vi "AOL Z Cal load-Load handler.vi"(11 "Loaded file":refnum<vi>) -> ()   [LabVIEW 2013]
uses:
  Typedefs/Which path.ctl
  Typedefs/Read Write Enum.ctl
  Typedefs/Functional global standard states.ctl
  Configuration code/Calibration/Globals/gl_Calibration globals.vi
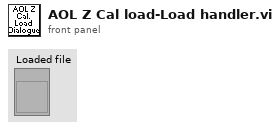
[diagram p1: front panel]
types:
  T1 = typedef "Which path.ctl" = enum16{"Configuration Files", "Calibration Files", "Images", "Setup.ini", "Loaded User profile.ini", "User's-Previous session.ini", "New user profile.ini", "Selected User profile.ini", "User profiles folder", "Power meter scaling.txt", "FOV Cal.ini"}
  T2 = typedef "Read Write Enum.ctl" = enum16{"Read", "Write"}
  T3 = typedef "Functional global standard states.ctl" = enum16{"Initialise", "Read", "Write", "Load", "Save", "Clear"}
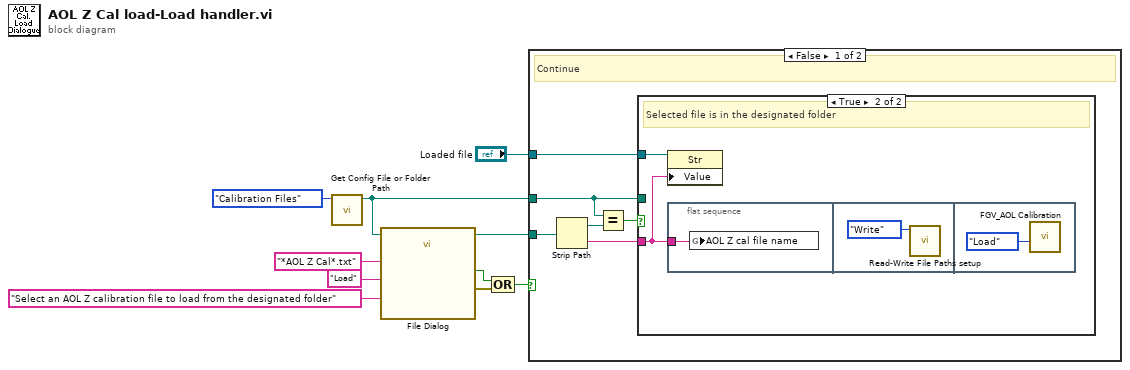
[diagram p0: block diagram]
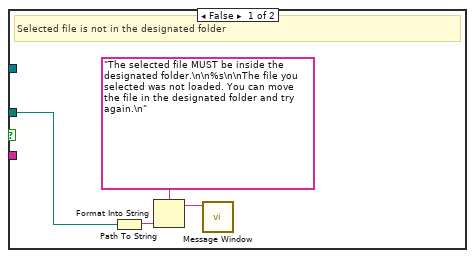
[diagram p2: hidden frame]
diagram:
  n1 = call "Get Config File or Folder Path.vi"("Which file or folder?"=Which_path."Calibration Files" ("Which file?")) -> ("File Path"=w2:path)  [unwired: 8 in, 2 out]
  n2 = call "File Dialog"("start path"=w2, "prompt"="Select an AOL Z calibration file to load from the designated folder", "button label"="Load", "pattern (all files)"="*AOL Z Cal*.txt") -> ("selected path"=w3:path, "cancelled"=w8:bool, "error out"=w7:errorcluster)  [unwired: 8 in, 1 out]
  n3 = Compound Arithmetic op=OR(w8, w7) -> (w6:bool)
  n4 = case shown="False" w6 {
    tunnel: w3 -> [w16 _]
    tunnel: w2 -> [w12 _]
    tunnel: "Loaded file" -> [w11 _]
    frame False {
      # "Continue"
      n5 = Strip Path(path=w16) -> (stripped path=w14:path, name=w15:string)
      n6 = Equal?(x=w12, y=w14) -> (x = y?=w13:bool)
      n7 = case shown="True" w13 {
        tunnel: w15 -> [_ w21]
        tunnel: w12 -> [w17 _]
        tunnel: w11 -> [_ w22]
        frame False {
          # "Selected file is not in the designated folder"
          n8 = Path To String(path=w17) -> (string=w18:string)
          n9 = Format Into String(format string="The selected file MUST be inside the designated folder.\n\n%s\n\nThe file you selected was not loaded. You can move the file in the designated folder and try again.\n" ("Message string"), w18) -> (resulting string=w19:string)  [unwired: 2 in, 1 out]
          n10 = call "Message Window.vi"("Message string"=w19) -> ()  [unwired: 10 in, 1 out]
        }
        frame True {
          # "Selected file is in the designated folder"
          n11 = property class="Str"(reference=w22, "Value"=w21) -> ()  [unwired: 1 in, 2 out]
          n12 = flat-sequence {
            tunnel: w21 -> [w23]
            frame #0 {
              n13 = global write "gl_Calibration globals.vi" "AOL Z cal file name"(w23) -> ()
            }
            frame #1 {
              n14 = call "Read-Write File Paths setup.vi"("Function"=Read_Write_Enum."Write") -> ()  [unwired: 10 in, 1 out]
            }
            frame #2 {
              n15 = call "FGV_AOL Calibration.vi"("Function"=Functional_global_standard_states."Load") -> ()  [unwired: 8 in, 3 out]
            }
          }
        }
      }
    }
    frame True {
      # "Cancelled or Error"
    }
  }
